vi "Set Sample Period.vi"(9 "Record?":bool, 10 "Storage Period (s)":dbl=0.1 min=0.001 format="%#_6p", 11 "Refresh Period (s)":dbl=0.1 min=0.001 format="%#_6p") -> (0 "Rate":dbl, 1 "times":i32[](array[numeric]), 2 "Acture Storage Period (s)":dbl=0.1 min=0.001 format="%#_6p", 3 "Acture Refresh Period (s)":dbl=0.1 min=0.001 format="%#_6p")   [LabVIEW 2018]
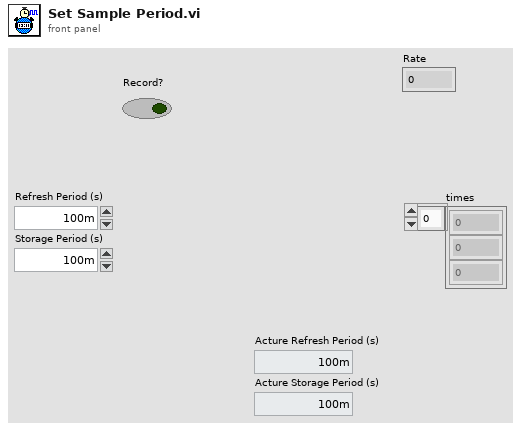
[diagram p1: front panel]
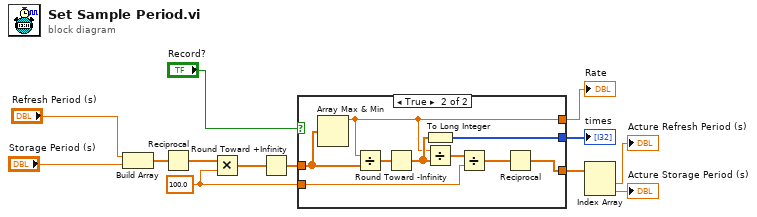
[diagram p0: block diagram]
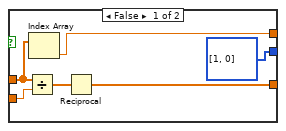
[diagram p2: hidden frame]
diagram:
  w6 = 100.0 ("y")
  n1 = Build Array("Refresh Period (s)", "Storage Period (s)") -> (w7:dbl[])
  n2 = Reciprocal(x=w7) -> (1/x=w8:dbl[])
  n3 = Multiply(x=w8, y=w6) -> (x*y=w5:dbl[])
  n4 = Round Toward +Infinity(x=w5) -> (ceil(x): smallest int >= x=w4:dbl[])
  n5 = case shown="True" "Record?" {
    tunnel: w6 -> [w16 w27]
    tunnel: [w15 w25] -> w3
    tunnel: w4 -> [w17 w22]
    tunnel: [w19 w21] -> w11
    tunnel: [i32[] [1, 0] w20] -> w2
    frame False {
      n6 = Divide(x=w17, y=w16) -> (x/y=w18:dbl[])
      n7 = Index Array(array=w17) -> (element=w19:dbl)  [unwired: 1 in]
      n8 = Reciprocal(x=w18) -> (1/x=w15:dbl[])
    }
    frame True {
      n9 = Array Max & Min(array=w22) -> (max value=w21:dbl)  [unwired: 3 out]
      n10 = Divide(x=w21, y=w22) -> (x/y=w28:dbl[])
      n11 = Round Toward -Infinity(1:w28) -> (0:w24:dbl[])
      n12 = To Long Integer(number=w24) -> (32bit integer=w20:i32[])
      n13 = Divide(x=w21, y=w24) -> (x/y=w23:dbl[])
      n14 = Divide(x=w23, y=w27) -> (x/y=w26:dbl[])
      n15 = Reciprocal(x=w26) -> (1/x=w25:dbl[])
    }
  }
  "times" <- w2
  "Rate" <- w11
  n16 = Index Array(array=w3) -> (element #1=→"Acture Refresh Period (s)":dbl, element #2=→"Acture Storage Period (s)":dbl)  [unwired: 2 in]
